vi "Motion_Profiling.vi"() -> ()   [LabVIEW 2016]
uses:
  <vilib>/Rock Robotics/WPI/Utilities/WPI_GetSetVariantRefNum.vi
panel:
  in  "Constants":T1={"kV"=0.0097, "kA"=0.0013, "Velocity PID"={"P"=0.03, "I"=0.0, "D"=0.0}, "Position PID"={"P"=0.0, "I"=0.0, "D"=0.0}}
  in  "Control mode":bool=TRUE
  in  "Max Speed":dbl=80.0 format="%#_13g"
  in  "Max Accel":dbl=180.0 format="%#_13g"
  in  "Max Jerk":dbl=200.0 format="%#_13g"
  in  "Motion Mode":bool=TRUE
  in  "DistanceR (in)":dbl=100.0
  in  "DistanceL (in)":dbl=120.0
  out "Position Chart":cluster{"pos":dbl, "pos":dbl}(graph)
  out "Velocity Chart":cluster{"vel":dbl, "vel":dbl}(graph)
  in  "Chart Slowing":u32(knob)=4 scale=1.0..10.0
  # "should probably be enums"
  # "Remember to make default!"
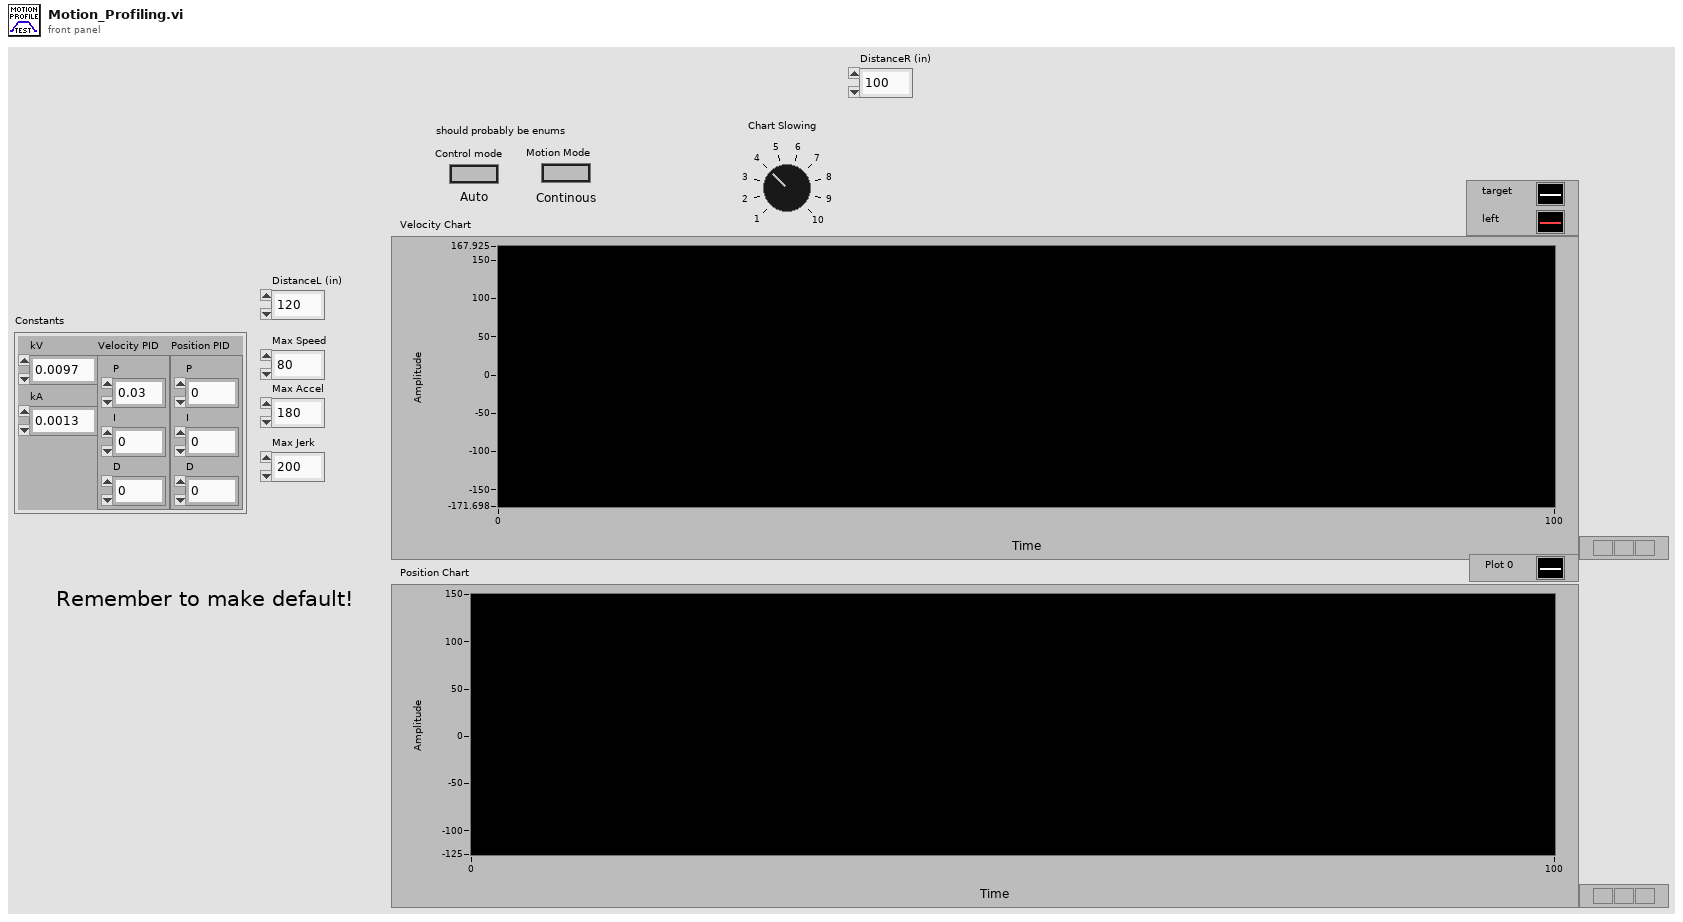
[diagram p1: front panel]
types:
  T1 = cluster{"kV":dbl, "kA":dbl, "Velocity PID":cluster{"P":dbl, "I":dbl, "D":dbl}, "Position PID":cluster{"P":dbl, "I":dbl, "D":dbl}}
  T2 = typedef "WPI_PotentiometerDevRef.ctl" = cluster{"DevStatus":errorcluster, "Analog Channel":T3, "Invert Output":bool}
  T3 = typedef "FPGA_AIChannel.ctl" = enum8{"AI 0", "AI 1", "AI 2", "AI 3", "AI MXP 0", "AI MXP 1", "AI MXP 2", "AI MXP 3", "Invalid"}
  T4 = typedef "WPI_JoystickDevRef.ctl" = cluster{"Device":T5}
  T5 = typedef "WPI_JoystickDeviceEnum.ctl" = enum16{"USB 0", "USB 1", "USB 2", "USB 3", "USB 4", "USB 5"}
  T6 = typedef "WPI_RobotDriveDevRef.ctl" = cluster{"DevStatus":errorcluster, "Motors[]":T7[], "Square Inputs":bool, "Max Output":dbl}
  T7 = typedef "WPI_MotorControlDeviceRef.ctl" = cluster{"DeviceStatus":errorcluster, "Type":T8, "PWM":cluster{"PWM Channel":T9, "DeadBand":T10}, "CAN":cluster{"Device Number":u8, "SetOutput VI Ref":variant, "GetOutput VI Ref":variant, "Enable VI Ref":variant, "Disable VI Ref":variant, "Data":variant}, "Invert":bool}
  T8 = typedef "WPI_MotorControlType.ctl" = enum16{"PWM", "CAN"}
  T9 = typedef "FPGA_DIOPWMChannel.ctl" = enum8{"PWM 0", "PWM 1", "PWM 2", "PWM 3", "PWM 4", "PWM 5", "PWM 6", "PWM 7", "PWM 8", "PWM 9", "PWM MXP 0", "PWM MXP 1", "PWM MXP 2", "PWM MXP 3", "PWM MXP 4", "PWM MXP 5", "PWM MXP 6", "PWM MXP 7", "PWM MXP 8", "PWM MXP 9", "Invalid"}
  T10 = typedef "WPI_PWMDeadband.ctl" = cluster{"Name":string, "maxPositivePwm":i32, "minPositivePwm":i32, "centerPwm":i32, "maxNegativePwm":i32, "minNegativePwm":i32, "angularRange":u16}
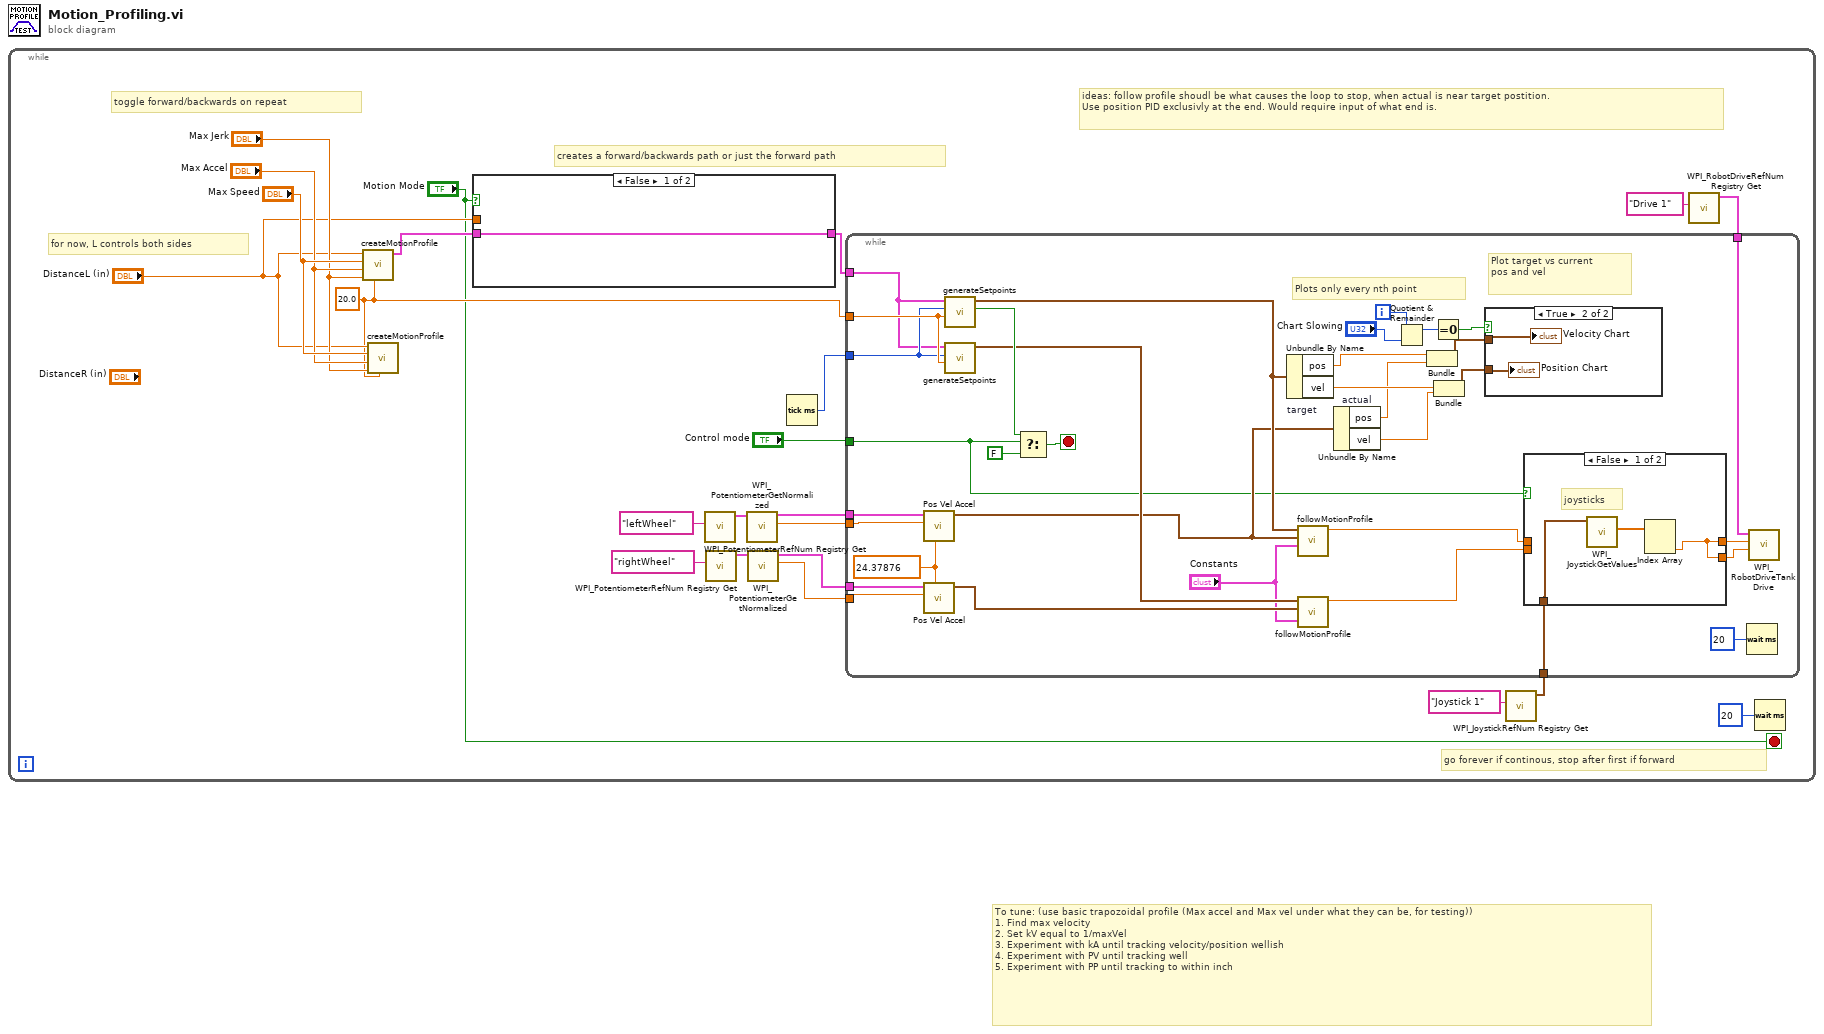
[diagram p0: block diagram]
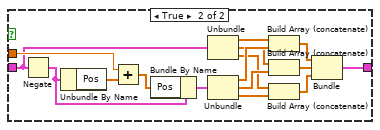
[diagram p2: hidden frame]
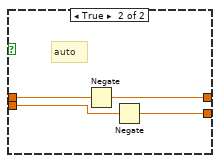
[diagram p3: hidden frame]
diagram:
  # "To tune: (use basic trapozoidal profile (Max accel and Max vel under what they can be, for testing))\n1. Find max velocity\n2. Set kV equal to 1/maxVel\n3. Experiment with kA until tracking velocity/position wellish\n4. Experiment with PV until tracking well\n5. Experiment with PP until tracking to within inch"
  n1 = while {
    stop <- "Motion Mode" stop-if-true
    w2 = 20.0 ("Motion Profile Control Frame Rate")
    # "ideas: follow profile shoudl be what causes the loop to stop, when actual is near target postition.\nUse position PID exclusivly at the end. Would require input of what end is."
    # "go forever if continous, stop after first if forward"
    # "creates a forward/backwards path or just the forward path"
    # "toggle forward/backwards on repeat"
    # "for now, L controls both sides"
    n2 = call "createMotionProfile.vi"("ms per frame"=w2, "Max Jerk (In/sec^3)"="Max Jerk", "Max Acceleration (In/sec^2)"="Max Accel", "Max Speed (In/sec)"="Max Speed", "Inches to Travel"="DistanceL (in)") -> ("Profile"=w5:cluster{"Pos":dbl[], "Vel":dbl[], "accel":dbl[]})  [unwired: 6 in]
    n3 = call "createMotionProfile.vi"("ms per frame"=w2, "Max Jerk (In/sec^3)"="Max Jerk", "Max Acceleration (In/sec^2)"="Max Accel", "Max Speed (In/sec)"="Max Speed", "Inches to Travel"="DistanceL (in)") -> ()  [unwired: 6 in, 1 out]
    n4 = case shown="False" "Motion Mode" {
      tunnel: w5 -> [w24 w35]
      tunnel: [w24 w28] -> w4
      tunnel: "DistanceL (in)" -> [_ w39]
      frame False {
      }
      frame True {
        n5 = Negate(x=w35) -> (-x=w37:cluster{"Pos":dbl[], "Vel":dbl[], "accel":dbl[]})
        n6 = Unbundle By Name(w37) -> ("Pos"=w40:dbl[])
        n7 = Add(x=w39, y=w40) -> (x+y=w38:dbl[])
        n8 = Bundle By Name(cluster=w37, "Pos"=w38) -> (w36:cluster{"Pos":dbl[], "Vel":dbl[], "accel":dbl[]})
        n9 = Unbundle(w35) -> ("Pos"=w34:dbl[], "Vel"=w32:dbl[], "accel"=w30:dbl[])
        n10 = Unbundle(w36) -> ("Pos"=w33:dbl[], "Vel"=w31:dbl[], "accel"=w29:dbl[])
        n11 = Build Array (concatenate)(w34, w33) -> (w27:dbl[])
        n12 = Build Array (concatenate)(w32, w31) -> (w26:dbl[])
        n13 = Build Array (concatenate)(w30, w29) -> (w25:dbl[])
        n14 = Bundle(w27, w26, w25) -> (w28:cluster{dbl[], dbl[], dbl[]})  [unwired: 1 in]
      }
    }
    n15 = call <vilib>:"WPI_PotentiometerRefNum Registry Get.vi"("refnum name"="leftWheel") -> ("PotDevRef"=w23:T2)  [unwired: 9 in, 1 out]
    n16 = call <vilib>:"WPI_PotentiometerRefNum Registry Get.vi"("refnum name"="rightWheel") -> ("PotDevRef"=w22:T2)  [unwired: 9 in, 1 out]
    n17 = call <vilib>:"WPI_PotentiometerGetNormalized.vi"("PotDevRef"=w23) -> ("Normalized Value"=w8:dbl, "PotDevRef"=w11:T2)  [unwired: 8 in, 1 out]
    n18 = call <vilib>:"WPI_PotentiometerGetNormalized.vi"("PotDevRef"=w22) -> ("Normalized Value"=w9:dbl, "PotDevRef"=w10:T2)  [unwired: 8 in, 1 out]
    n19 = Tick Count (ms)() -> (millisecond timer value=w16:u32)
    n20 = call <vilib>:"WPI_JoystickRefNum Registry Get.vi"("refnum name"="Joystick 1") -> ("JoystickDevRef"=w13:T4)  [unwired: 9 in, 1 out]
    n21 = call <vilib>:"WPI_RobotDriveRefNum Registry Get.vi"("refnum name"="Drive 1") -> ("RobotDriveDevRef"=w6:T6)  [unwired: 9 in, 1 out]
    n22 = while {
      tunnel: w4 -> [w61]
      tunnel: w2 -> [w63]
      tunnel: w16 -> [w62]
      tunnel: w13 -> [w45]
      tunnel: "Control mode" -> [w48]
      tunnel: w11 -> [w58]
      tunnel: w10 -> [w57]
      tunnel: w9 -> [w56]
      tunnel: w8 -> [w55]
      tunnel: w6 -> [w42]
      i -> [w74]
      stop <- w73 stop-if-true
      w59 = 24.37876 ("distance/rotation")
      # "Plot target vs current\npos and vel"
      # "Plots only every nth point"
      n23 = call "Pos Vel Accel.vi"("distance/rotation"=w59, "Starting pot value"=w55, "PotDevRef"=w58) -> ("Current Values"=w51:cluster{"pos":dbl, "vel":dbl, "accel":dbl})  [unwired: 8 in]
      n24 = call "Pos Vel Accel.vi"("distance/rotation"=w59, "Starting pot value"=w56, "PotDevRef"=w57) -> ("Current Values"=w60:cluster{"pos":dbl, "vel":dbl, "accel":dbl})  [unwired: 8 in]
      n25 = call "generateSetpoints.vi"("ms/frame"=w63, "start time"=w62, "Profile"=w61) -> ("Done?"=w70:bool, "Setpoint"=w54:cluster{"pos":dbl, "vel":dbl, "accel":dbl})  [unwired: 7 in]
      n26 = call "generateSetpoints.vi"("ms/frame"=w63, "start time"=w62, "Profile"=w61) -> ("Setpoint"=w64:cluster{"pos":dbl, "vel":dbl, "accel":dbl})  [unwired: 7 in, 1 out]
      n27 = Select(t=w70, s=w48, f=FALSE) -> (s? t:f=w73:bool)
      n28 = Unbundle By Name "target"(w54) -> ("pos"=w53:dbl, "vel"=w52:dbl)
      n29 = call "followMotionProfile.vi"("Constants"="Constants", "Feedback"=w51, "Target"=w54) -> ("Duty Cycle"=w47:dbl)  [unwired: 8 in]
      n30 = call "followMotionProfile.vi"("Constants"="Constants", "Feedback"=w60, "Target"=w64) -> ("Duty Cycle"=w46:dbl)  [unwired: 8 in]
      n31 = Unbundle By Name "actual"(w51) -> ("pos"=w50:dbl, "vel"=w49:dbl)
      n32 = Quotient & Remainder(x=w74, y="Chart Slowing") -> (x-y*floor(x/y)=w69:u32)  [unwired: 1 out]
      n33 = Bundle("pos"=w53, "pos"=w50) -> (w65:cluster{"pos":dbl, "pos":dbl})  [unwired: 1 in]
      n34 = Equal To 0?(x=w69) -> (x = 0?=w68:bool)
      n35 = Bundle("vel"=w52, "vel"=w49) -> (w66:cluster{"vel":dbl, "vel":dbl})  [unwired: 1 in]
      n36 = case shown="True" w68 {
        tunnel: w66 -> [_ w82]
        tunnel: w65 -> [_ w83]
        frame False {
        }
        frame True {
          "Velocity Chart" <- w83
          "Position Chart" <- w82
        }
      }
      n37 = case shown="False" w48 {
        tunnel: w46 -> [_ w81]
        tunnel: w47 -> [_ w80]
        tunnel: w45 -> [w76 _]
        tunnel: [w75 w79] -> w43
        tunnel: [w75 w78] -> w44
        frame False {
          # "joysticks"
          n38 = call <vilib>:"WPI_JoystickGetValues.vi"("JoystickDevRef"=w76) -> ("Axes"=w77:dbl[])  [unwired: 6 in, 4 out]
          n39 = Index Array(array=w77) -> (element #2=w75:dbl)  [unwired: 2 in, 1 out]
        }
        frame True {
          # "auto"
          n40 = Negate(x=w80) -> (-x=w79:dbl)
          n41 = Negate(x=w81) -> (-x=w78:dbl)
        }
      }
      n42 = Wait (ms)(milliseconds to wait=u32 20) -> ()  [unwired: 1 out]
      n43 = call <vilib>:"WPI_RobotDriveTankDrive.vi"("Right axis value"=w44, "Left axis value"=w43, "RobotDriveDevRef"=w42) -> ()  [unwired: 6 in, 3 out]
    }
    n44 = Wait (ms)(milliseconds to wait=u32 20) -> ()  [unwired: 1 out]
  }
